vi "set Tname.vi"(8 "error in (no error)":errorcluster caption="Fehler (Eingang, kein Fehler)", 10 "name":string, 11 "Test (Eingang)":refnum<class "Test.lvclass">) -> (0 "error out":errorcluster caption="Fehler (Ausgang)", 3 "Test (Ausgang)":refnum<class "Test.lvclass">)   [LabVIEW 2013, in "DatenKlassen.lvlib" / "Test.lvclass"]
uses:
  Test.lvclass
  Test.lvclass/Test.ctl
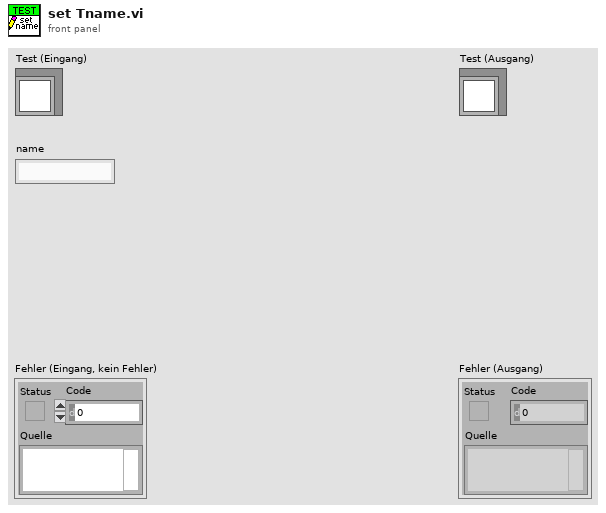
[diagram p1: front panel]
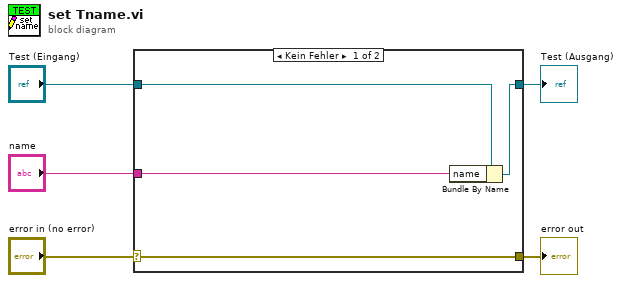
[diagram p0: block diagram]
diagram:
  n1 = case shown="Kein Fehler" "error in (no error)" {
    selector: "error in (no error)" -> [w9 w10]
    tunnel: [w9 w10] -> w4
    tunnel: [w7 w11] -> w2
    tunnel: "Test (Eingang)" -> [w8 w11]
    tunnel: "name" -> [w6 _]
    frame No Error {
      n2 = Bundle By Name(cluster=w8, "name"=w6) -> (w7:refnum<class "Test.lvclass">)
    }
    frame Error {
    }
  }
  "error out" <- w4
  "Test (Ausgang)" <- w2
